vi "zmq atomic counter destroy.vi"(8 "error in (no error)":errorcluster, 11 "counter_p_":u32) -> (0 "error out":errorcluster, 3 "counter_p_ out":u32)   [LabVIEW 2025, in "libzmq-v143-mt-4_3_6.lvlib"]
doc: "ZMQ_EXPORT void zmq_atomic_counter_destroy (void **counter_p_);"
uses:
  libzmq-v143-mt-4_3_6.lvlib
  LV/LibZMQ/libzmq/lv_x86/bin/Release/libzmq-v143-mt-4_3_6.dll
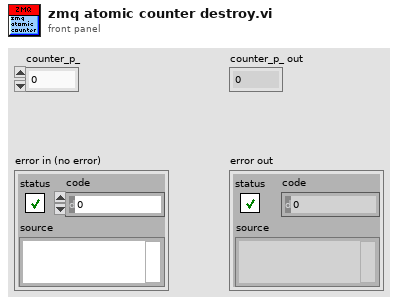
[diagram p1: front panel]
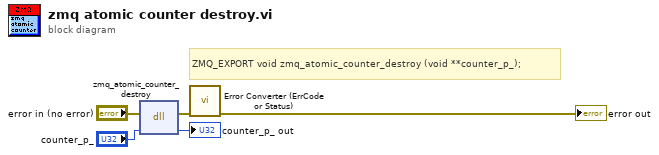
[diagram p0: block diagram]
diagram:
  # "ZMQ_EXPORT void zmq_atomic_counter_destroy (void **counter_p_);"
  n1 = dll-call lib="C:/LV/LibZMQ/libzmq/lv_x86/bin/Release/libzmq-v143-mt-4_3_6.*" fn="zmq_atomic_counter_destroy"(error in="error in (no error)", "counter_p_"="counter_p_") -> (error out=w2:errorcluster, "counter_p_"=→"counter_p_ out":u32)  [unwired: 3 in, 1 out]
  n2 = call "Error Converter (ErrCode or Status).vi"("error in (no error)"=w2) -> ("error out"=→"error out":errorcluster)  [unwired: 10 in]
